vi "New Report.vi"(2 "error in (no error)":errorcluster, 3 "Output Path":path, 4 "Source Path":path) -> (0 "error out":errorcluster, 1 "Report Ref":T1)   [LabVIEW 2013, in "XCel Report Engine.lvlib"]
doc: "Creates a new XCelReportEngine report session from an existing Excel workbook or template.\n\nThe source file must be an OpenXML Excel workbook or template in XLSX or XLTX format. The source file is opened through an internal working copy and is not modified.\n\nOutput Path specifies the XLSX file that will be created when the report is saved. An existing output file can be overwritten.\n\nThe returned Report Ref identifies the open report session and must be passed unchanged to subsequent report operations. Close the session with Close Report.vi when report generation is complete.\n\nThis VI does not require Microsoft Excel or Microsoft Office."
uses:
  XCel Report Engine.lvlib
  Controls/Report Ref.ctl
  C:/Users/m.santucci/Documents/ChatGPT/LV_REPORT_ENGINE/LV/DotNet/XCelReportEngine.dll
  LV/DotNet/XCelReportEngine.dll
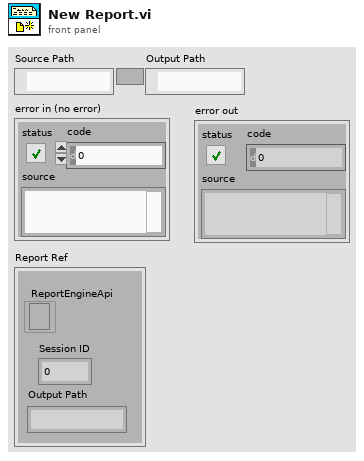
[diagram p1: front panel]
types:
  T1 = typedef "XCel Report Engine.lvlib/Report Ref.ctl" = cluster{"Session ID":i32, "Output Path":string, "ReportEngineApi":refnum<k24>}
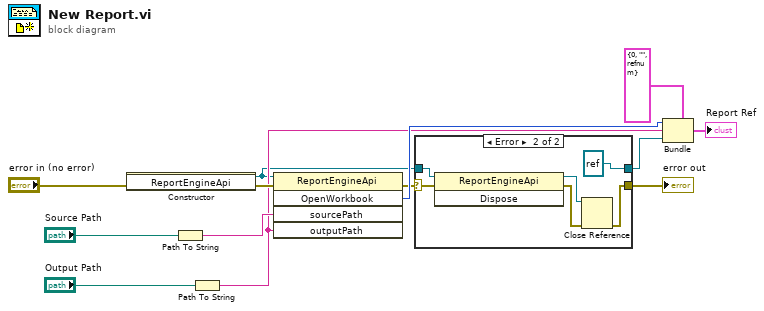
[diagram p0: block diagram]
diagram:
  n1 = constructor class="ReportEngineApi"(error in="error in (no error)") -> (reference out=w4:refnum<k24>, error out=w8:errorcluster)  [unwired: 2 in, 1 out]
  n2 = Path To String(path="Source Path") -> (string=w11:string)
  n3 = Path To String(path="Output Path") -> (string=w6:string)
  n4 = invoke class="ReportEngineApi" method="OpenWorkbook"(reference=w4, error in=w8, "sourcePath"=w11, "outputPath"=w6) -> (error out=w5:errorcluster, "OpenWorkbook"=w7:i32)  [unwired: 1 in, 3 out]
  n5 = case shown="Error" w5 {
    selector: w5 -> [w15 w18]
    tunnel: w4 -> [w14 w21]
    tunnel: [w15 w17] -> w3
    tunnel: [w14 refnum<k24> refnum ("new reference")] -> w1
    frame No Error {
    }
    frame Error {
      n6 = invoke class="ReportEngineApi" method="Dispose"(reference=w21, error in=w18) -> (reference out=w20:refnum<k24>, error out=w19:errorcluster)  [unwired: 1 in, 1 out]
      n7 = Close Reference(reference=w20, error in (no error)=w19) -> (error out=w17:errorcluster)
    }
  }
  "error out" <- w3
  n8 = Bundle(cluster=T1 {"Session ID"=0, "Output Path"="", "ReportEngineApi"=refnum} ("Report Ref"), "Session ID"=w7, "Output Path"=w6, "ReportEngineApi"=w1) -> (→"Report Ref":T1)
